vi "传感器特性判定.vi"(7 "Result":refnum<vi>, 10 "判定参数":T1, 11 "XY曲线":cluster{"X":dbl[], "Y":dbl[]}[](array[cluster])) -> (2 "判定项长度":i32, 3 "OK？":bool)   [LabVIEW 2020]
uses:
  <vilib>/Analysis/6fits.llb/Curve Fitting Criteria.ctl
  <vilib>/Analysis/NI_AALPro.lvlib
  <vilib>/Analysis/NI_AAL_Geometry.lvlib
panel:
  out "定点设置":dbl
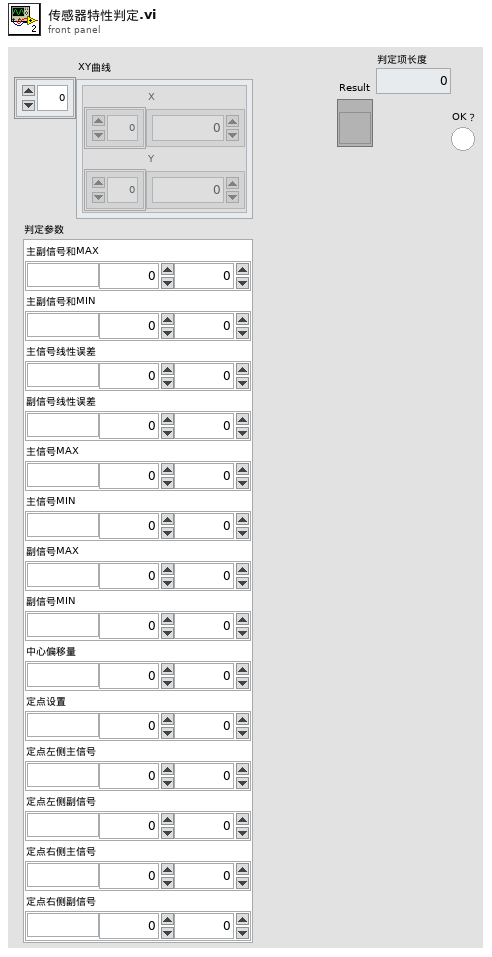
[diagram p1: front panel]
types:
  T1 = cluster{"主副信号和MAX":cluster{"单位":string, "下限":dbl, "上限":dbl}, "主副信号和MIN":cluster{"单位":string, "下限":dbl, "上限":dbl}, "主信号线性误差":cluster{"单位":string, "下限":dbl, "上限":dbl}, "副信号线性误差":cluster{"单位":string, "下限":dbl, "上限":dbl}, "主信号MAX":cluster{"单位":string, "下限":dbl, "上限":dbl}, "主信号MIN":cluster{"单位":string, "下限":dbl, "上限":dbl}, "副信号MAX":cluster{"单位":string, "下限":dbl, "上限":dbl}, "副信号MIN":cluster{"单位":string, "下限":dbl, "上限":dbl}, "中心偏移量":cluster{"单位":string, "下限":dbl, "上限":dbl}, "定点设置":cluster{"单位":string, "下限":dbl, "上限":dbl}, "定点左侧主信号":cluster{"单位":string, "下限":dbl, "上限":dbl}, "定点左侧副信号":cluster{"单位":string, "下限":dbl, "上限":dbl}, "定点右侧主信号":cluster{"单位":string, "下限":dbl, "上限":dbl}, "定点右侧副信号":cluster{"单位":string, "下限":dbl, "上限":dbl}}
  T2 = typedef "NI_AALPro.lvlib/Curve Fitting Criteria.ctl" = u16
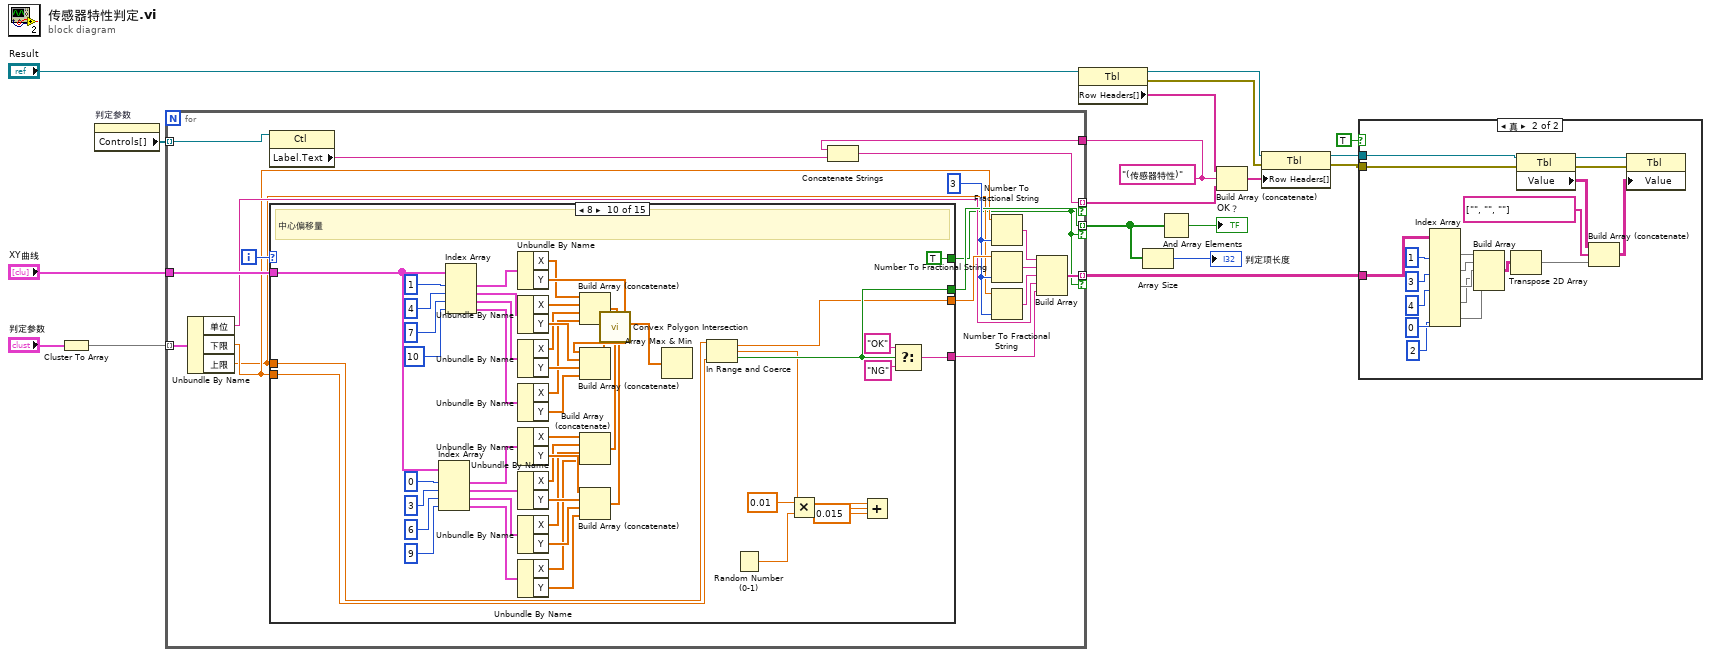
[diagram p0: block diagram]
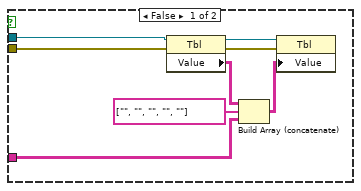
[diagram p2: hidden frame]
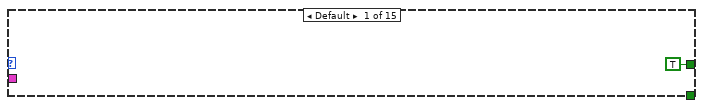
[diagram p3: hidden frame]
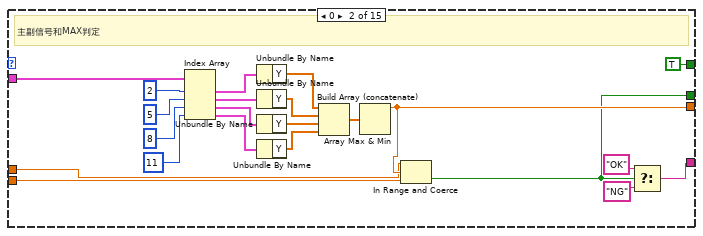
[diagram p4: hidden frame]
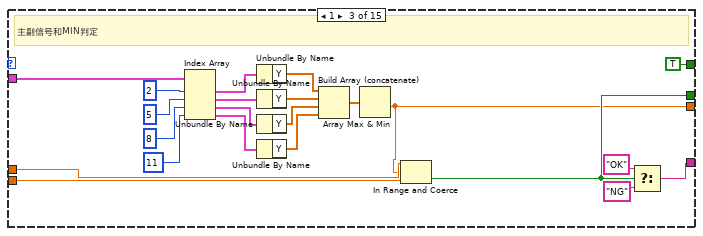
[diagram p5: hidden frame]
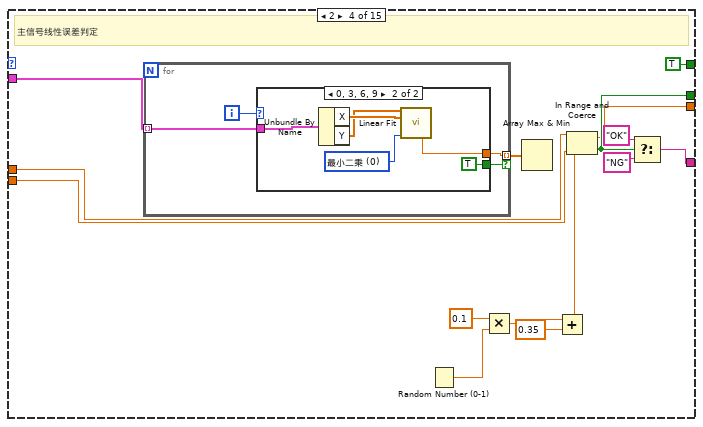
[diagram p6: hidden frame]
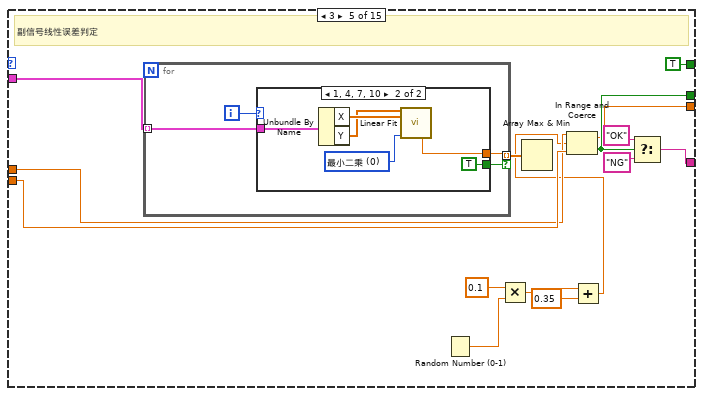
[diagram p8: hidden frame]
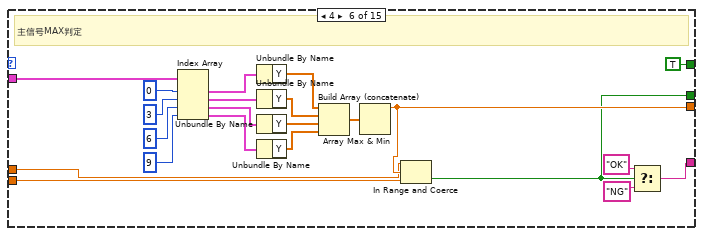
[diagram p10: hidden frame]
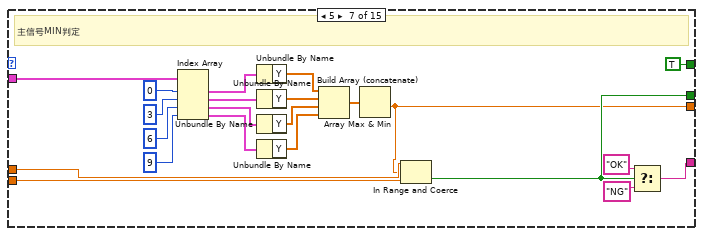
[diagram p11: hidden frame]
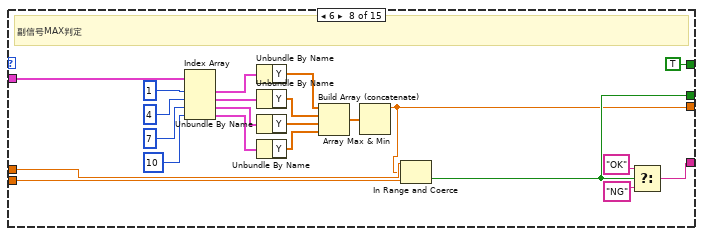
[diagram p12: hidden frame]
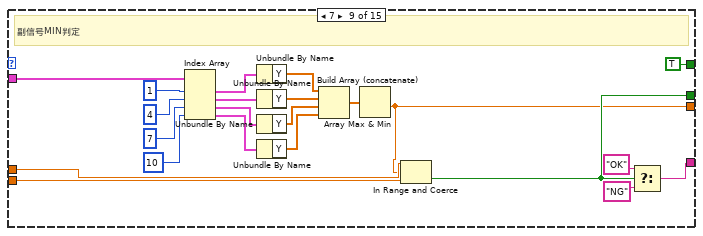
[diagram p13: hidden frame]
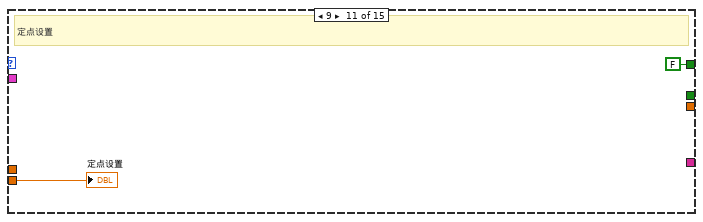
[diagram p14: hidden frame]
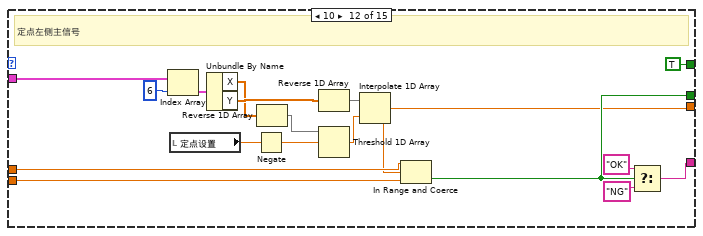
[diagram p15: hidden frame]
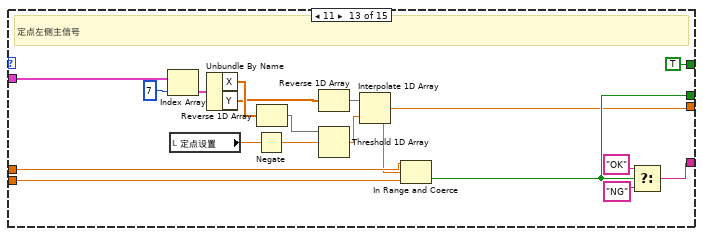
[diagram p16: hidden frame]
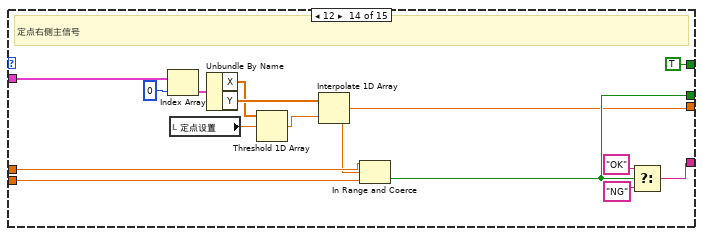
[diagram p17: hidden frame]
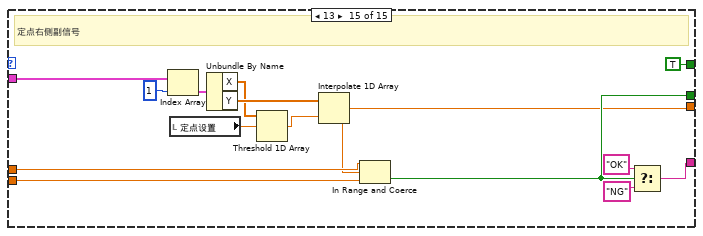
[diagram p18: hidden frame]
diagram:
  w1 = "(传感器特性)" ("Label.Text")
  n1 = Cluster To Array(cluster="判定参数") -> (array=w18:cluster{"单位":string, "下限":dbl, "上限":dbl}[])
  n2 = property on="判定参数" class="Clust (严格)"() -> ("Controls[]"=w16:refnum<vi>[])  [unwired: 2 in, 2 out]
  n3 = for {
    tunnel: w18 -> [w37] mode=indexing
    tunnel: w16 -> [w35] mode=indexing
    tunnel: "XY曲线" -> [w33]
    tunnel: [w27] -> w3 mode=indexing if=w21
    tunnel: [w23] -> w5 mode=indexing if=w21
    tunnel: [w20] -> w8 mode=indexing if=w21
    tunnel: w1 -> [w19]
    i -> [w36]
    w32 = i16 3 ("精度(6)")
    n4 = Unbundle By Name(w37) -> ("单位"=w26:string, "下限"=w25:dbl, "上限"=w24:dbl)
    n5 = property class="Ctl"(reference=w35) -> ("Label.Text"=w22:string)  [unwired: 1 in, 2 out]
    n6 = case shown="8" w36 {
      tunnel: [_ w46 w61 w84 w109 w140 w156 w178 w200 w222 _ w278 w295 w312 w327] -> w34
      tunnel: w33 -> [_ w60 w82 w90 w115 w154 w176 w198 w220 w240 _ w291 w309 w324 w339]
      tunnel: [_ w43 w66 w95 w120 w137 w160 w182 w204 w257 _ w287 w305 w320 w335] -> w28
      tunnel: [_ w42 w65 w94 w119 w136 w159 w181 w203 w256 _ w286 w304 w319 w334] -> w27
      tunnel: w25 -> [_ w41 w64 w93 w118 w135 w158 w180 w202 w255 w272 w285 w303 w318 w333]
      tunnel: w24 -> [_ w40 w63 w92 w117 w134 w157 w179 w201 w254 _ w284 w302 w317 w332]
      tunnel: [TRUE TRUE TRUE TRUE TRUE TRUE TRUE TRUE TRUE TRUE FALSE TRUE TRUE TRUE TRUE] -> w21
      frame Default {
      }
      frame 0 {
        # "主副信号和MAX判定"
        n7 = Index Array(array=w60, index #1=2 ("索引"), index #2=5 ("索引"), index #3=8 ("索引"), index #4=11 ("索引")) -> (element #1=w55:cluster{"X":dbl[], "Y":dbl[]}, element #2=w52:cluster{"X":dbl[], "Y":dbl[]}, element #3=w53:cluster{"X":dbl[], "Y":dbl[]}, element #4=w54:cluster{"X":dbl[], "Y":dbl[]})
        n8 = Unbundle By Name(w55) -> ("Y"=w51:dbl[])
        n9 = Unbundle By Name(w52) -> ("Y"=w50:dbl[])
        n10 = Unbundle By Name(w53) -> ("Y"=w49:dbl[])
        n11 = Unbundle By Name(w54) -> ("Y"=w48:dbl[])
        n12 = Build Array (concatenate)(w51, w50, w49, w48) -> (w47:dbl[])
        n13 = Array Max & Min(array=w47) -> (max value=w46:dbl)  [unwired: 3 out]
        n14 = In Range and Coerce(upper limit=w40, x=w46, lower limit=w41) -> (In Range?=w42:bool)  [unwired: 1 out]
        n15 = Select(t="OK", s=w42, f="NG") -> (s? t:f=w43:string)
      }
      frame 1 {
        # "主副信号和MIN判定"
        n16 = Index Array(array=w82, index #1=2 ("索引"), index #2=5 ("索引"), index #3=8 ("索引"), index #4=11 ("索引")) -> (element #1=w77:cluster{"X":dbl[], "Y":dbl[]}, element #2=w74:cluster{"X":dbl[], "Y":dbl[]}, element #3=w75:cluster{"X":dbl[], "Y":dbl[]}, element #4=w76:cluster{"X":dbl[], "Y":dbl[]})
        n17 = Unbundle By Name(w77) -> ("Y"=w73:dbl[])
        n18 = Unbundle By Name(w74) -> ("Y"=w72:dbl[])
        n19 = Unbundle By Name(w75) -> ("Y"=w71:dbl[])
        n20 = Unbundle By Name(w76) -> ("Y"=w70:dbl[])
        n21 = Build Array (concatenate)(w73, w72, w71, w70) -> (w69:dbl[])
        n22 = Array Max & Min(array=w69) -> (min value=w61:dbl)  [unwired: 3 out]
        n23 = In Range and Coerce(upper limit=w63, x=w61, lower limit=w64) -> (In Range?=w65:bool)  [unwired: 1 out]
        n24 = Select(t="OK", s=w65, f="NG") -> (s? t:f=w66:string)
      }
      frame 2 {
        # "主信号线性误差判定"
        n25 = for {
          tunnel: w90 -> [w100] mode=indexing
          tunnel: [w99] -> w89 mode=indexing if=w98
          i -> [w101]
          n26 = case shown="0, 3, 6, 9" w101 {
            tunnel: w100 -> [_ w107]
            tunnel: [_ w105] -> w99
            tunnel: [_ TRUE] -> w98
            frame Default {
            }
            frame 0, 3, 6, 9 {
              w106 = T2 0 items=["最小二乘", "最小绝对残差", "Bisquare"] ("method")
              n27 = Unbundle By Name(w107) -> ("X"=w103:dbl[], "Y"=w102:dbl[])
              n28 = call <vilib>:"Linear Fit.vi"("Y"=w102, "X"=w103, "method"=w106) -> ("residue"=w105:dbl)  [unwired: 8 in, 4 out]
            }
          }
        }
        n29 = Random Number (0-1)() -> (number: 0 to 1=w87:dbl)
        n30 = Multiply(x=0.1, y=w87) -> (x*y=w86:dbl)
        n31 = Array Max & Min(array=w89) -> ()  [unwired: 4 out]
        n32 = Add(x=w86, y=0.35) -> (x+y=w83:dbl)
        n33 = In Range and Coerce(upper limit=w92, x=w83, lower limit=w93) -> (coerced(x)=w84:dbl, In Range?=w94:bool)
        n34 = Select(t="OK", s=w94, f="NG") -> (s? t:f=w95:string)
      }
      frame 3 {
        # "副信号线性误差判定"
        n35 = for {
          tunnel: w115 -> [w125] mode=indexing
          tunnel: [w124] -> w114 mode=indexing if=w123
          i -> [w126]
          n36 = case shown="1, 4, 7, 10" w126 {
            tunnel: w125 -> [_ w132]
            tunnel: [_ w130] -> w124
            tunnel: [_ TRUE] -> w123
            frame Default {
            }
            frame 1, 4, 7, 10 {
              w131 = T2 0 items=["最小二乘", "最小绝对残差", "Bisquare"] ("method")
              n37 = Unbundle By Name(w132) -> ("X"=w128:dbl[], "Y"=w127:dbl[])
              n38 = call <vilib>:"Linear Fit.vi"("Y"=w127, "X"=w128, "method"=w131) -> ("residue"=w130:dbl)  [unwired: 8 in, 4 out]
            }
          }
        }
        n39 = Random Number (0-1)() -> (number: 0 to 1=w113:dbl)
        n40 = Multiply(x=0.1, y=w113) -> (x*y=w112:dbl)
        n41 = Array Max & Min(array=w114) -> ()  [unwired: 4 out]
        n42 = Add(x=w112, y=0.35) -> (x+y=w108:dbl)
        n43 = In Range and Coerce(upper limit=w117, x=w108, lower limit=w118) -> (coerced(x)=w109:dbl, In Range?=w119:bool)
        n44 = Select(t="OK", s=w119, f="NG") -> (s? t:f=w120:string)
      }
      frame 4 {
        # "主信号MAX判定"
        n45 = Index Array(array=w154, index #1=0 ("索引"), index #2=3 ("索引"), index #3=6 ("索引"), index #4=9 ("索引")) -> (element #1=w149:cluster{"X":dbl[], "Y":dbl[]}, element #2=w146:cluster{"X":dbl[], "Y":dbl[]}, element #3=w147:cluster{"X":dbl[], "Y":dbl[]}, element #4=w148:cluster{"X":dbl[], "Y":dbl[]})
        n46 = Unbundle By Name(w149) -> ("Y"=w145:dbl[])
        n47 = Unbundle By Name(w146) -> ("Y"=w144:dbl[])
        n48 = Unbundle By Name(w147) -> ("Y"=w143:dbl[])
        n49 = Unbundle By Name(w148) -> ("Y"=w142:dbl[])
        n50 = Build Array (concatenate)(w145, w144, w143, w142) -> (w141:dbl[])
        n51 = Array Max & Min(array=w141) -> (max value=w140:dbl)  [unwired: 3 out]
        n52 = In Range and Coerce(upper limit=w134, x=w140, lower limit=w135) -> (In Range?=w136:bool)  [unwired: 1 out]
        n53 = Select(t="OK", s=w136, f="NG") -> (s? t:f=w137:string)
      }
      frame 5 {
        # "主信号MIN判定"
        n54 = Index Array(array=w176, index #1=0 ("索引"), index #2=3 ("索引"), index #3=6 ("索引"), index #4=9 ("索引")) -> (element #1=w171:cluster{"X":dbl[], "Y":dbl[]}, element #2=w168:cluster{"X":dbl[], "Y":dbl[]}, element #3=w169:cluster{"X":dbl[], "Y":dbl[]}, element #4=w170:cluster{"X":dbl[], "Y":dbl[]})
        n55 = Unbundle By Name(w171) -> ("Y"=w167:dbl[])
        n56 = Unbundle By Name(w168) -> ("Y"=w166:dbl[])
        n57 = Unbundle By Name(w169) -> ("Y"=w165:dbl[])
        n58 = Unbundle By Name(w170) -> ("Y"=w164:dbl[])
        n59 = Build Array (concatenate)(w167, w166, w165, w164) -> (w163:dbl[])
        n60 = Array Max & Min(array=w163) -> (min value=w156:dbl)  [unwired: 3 out]
        n61 = In Range and Coerce(upper limit=w157, x=w156, lower limit=w158) -> (In Range?=w159:bool)  [unwired: 1 out]
        n62 = Select(t="OK", s=w159, f="NG") -> (s? t:f=w160:string)
      }
      frame 6 {
        # "副信号MAX判定"
        n63 = Index Array(array=w198, index #1=1 ("索引"), index #2=4 ("索引"), index #3=7 ("索引"), index #4=10 ("索引")) -> (element #1=w193:cluster{"X":dbl[], "Y":dbl[]}, element #2=w190:cluster{"X":dbl[], "Y":dbl[]}, element #3=w191:cluster{"X":dbl[], "Y":dbl[]}, element #4=w192:cluster{"X":dbl[], "Y":dbl[]})
        n64 = Unbundle By Name(w193) -> ("Y"=w189:dbl[])
        n65 = Unbundle By Name(w190) -> ("Y"=w188:dbl[])
        n66 = Unbundle By Name(w191) -> ("Y"=w187:dbl[])
        n67 = Unbundle By Name(w192) -> ("Y"=w186:dbl[])
        n68 = Build Array (concatenate)(w189, w188, w187, w186) -> (w185:dbl[])
        n69 = Array Max & Min(array=w185) -> (max value=w178:dbl)  [unwired: 3 out]
        n70 = In Range and Coerce(upper limit=w179, x=w178, lower limit=w180) -> (In Range?=w181:bool)  [unwired: 1 out]
        n71 = Select(t="OK", s=w181, f="NG") -> (s? t:f=w182:string)
      }
      frame 7 {
        # "副信号MIN判定"
        n72 = Index Array(array=w220, index #1=1 ("索引"), index #2=4 ("索引"), index #3=7 ("索引"), index #4=10 ("索引")) -> (element #1=w215:cluster{"X":dbl[], "Y":dbl[]}, element #2=w212:cluster{"X":dbl[], "Y":dbl[]}, element #3=w213:cluster{"X":dbl[], "Y":dbl[]}, element #4=w214:cluster{"X":dbl[], "Y":dbl[]})
        n73 = Unbundle By Name(w215) -> ("Y"=w211:dbl[])
        n74 = Unbundle By Name(w212) -> ("Y"=w210:dbl[])
        n75 = Unbundle By Name(w213) -> ("Y"=w209:dbl[])
        n76 = Unbundle By Name(w214) -> ("Y"=w208:dbl[])
        n77 = Build Array (concatenate)(w211, w210, w209, w208) -> (w207:dbl[])
        n78 = Array Max & Min(array=w207) -> (min value=w200:dbl)  [unwired: 3 out]
        n79 = In Range and Coerce(upper limit=w201, x=w200, lower limit=w202) -> (In Range?=w203:bool)  [unwired: 1 out]
        n80 = Select(t="OK", s=w203, f="NG") -> (s? t:f=w204:string)
      }
      frame 8 {
        # "中心偏移量"
        n81 = Index Array(array=w240, index #1=0 ("索引"), index #2=3 ("索引"), index #3=6 ("索引"), index #4=9 ("索引")) -> (element #1=w267:cluster{"X":dbl[], "Y":dbl[]}, element #2=w264:cluster{"X":dbl[], "Y":dbl[]}, element #3=w265:cluster{"X":dbl[], "Y":dbl[]}, element #4=w266:cluster{"X":dbl[], "Y":dbl[]})
        n82 = Index Array(array=w240, index #1=1 ("索引"), index #2=4 ("索引"), index #3=7 ("索引"), index #4=10 ("索引")) -> (element #1=w245:cluster{"X":dbl[], "Y":dbl[]}, element #2=w248:cluster{"X":dbl[], "Y":dbl[]}, element #3=w247:cluster{"X":dbl[], "Y":dbl[]}, element #4=w246:cluster{"X":dbl[], "Y":dbl[]})
        n83 = Unbundle By Name(w245) -> ("X"=w239:dbl[], "Y"=w249:dbl[])
        n84 = Unbundle By Name(w248) -> ("X"=w238:dbl[], "Y"=w250:dbl[])
        n85 = Unbundle By Name(w247) -> ("X"=w237:dbl[], "Y"=w251:dbl[])
        n86 = Unbundle By Name(w246) -> ("X"=w236:dbl[], "Y"=w252:dbl[])
        n87 = Unbundle By Name(w267) -> ("X"=w235:dbl[], "Y"=w263:dbl[])
        n88 = Unbundle By Name(w264) -> ("X"=w234:dbl[], "Y"=w262:dbl[])
        n89 = Unbundle By Name(w265) -> ("X"=w233:dbl[], "Y"=w261:dbl[])
        n90 = Unbundle By Name(w266) -> ("X"=w232:dbl[], "Y"=w260:dbl[])
        n91 = Build Array (concatenate)(w239, w238, w237, w236) -> (w229:dbl[])
        n92 = Build Array (concatenate)(w249, w250, w251, w252) -> (w231:dbl[])
        n93 = Build Array (concatenate)(w235, w234, w233, w232) -> (w228:dbl[])
        n94 = Build Array (concatenate)(w263, w262, w261, w260) -> (w227:dbl[])
        n95 = call <vilib>:"Convex Polygon Intersection.vi"("Y 2"=w227, "X 2"=w228, "Y 1"=w231, "X 1"=w229) -> ("Intersection Y"=w230:dbl[])  [unwired: 5 in, 2 out]
        n96 = Array Max & Min(array=w230) -> ()  [unwired: 4 out]
        n97 = Random Number (0-1)() -> (number: 0 to 1=w225:dbl)
        n98 = Multiply(x=0.01, y=w225) -> (x*y=w224:dbl)
        n99 = Add(x=w224, y=0.015) -> (x+y=w221:dbl)
        n100 = In Range and Coerce(upper limit=w254, x=w221, lower limit=w255) -> (coerced(x)=w222:dbl, In Range?=w256:bool)
        n101 = Select(t="OK", s=w256, f="NG") -> (s? t:f=w257:string)
      }
      frame 9 {
        # "定点设置"
        "定点设置" <- w272
      }
      frame 10 {
        # "定点左侧主信号"
        n102 = Index Array(array=w291, index=6 ("索引")) -> (element=w290:cluster{"X":dbl[], "Y":dbl[]})
        n103 = local read "定点设置"() -> (w280:dbl)
        n104 = Unbundle By Name(w290) -> ("X"=w277:dbl[], "Y"=w279:dbl[])
        n105 = Negate(x=w280) -> (-x=w276:dbl)
        n106 = Reverse 1D Array(array=w277) -> (reversed array=w275:dbl[])
        n107 = Reverse 1D Array(array=w279) -> (reversed array=w274:dbl[])
        n108 = Threshold 1D Array(2:w276, 3:w275) -> (0:w281:dbl)  [unwired: 1 in]
        n109 = Interpolate 1D Array(1:w281, 2:w274) -> (0:w278:dbl)
        n110 = In Range and Coerce(upper limit=w284, x=w278, lower limit=w285) -> (In Range?=w286:bool)  [unwired: 1 out]
        n111 = Select(t="OK", s=w286, f="NG") -> (s? t:f=w287:string)
      }
      frame 11 {
        # "定点左侧主信号"
        n112 = Index Array(array=w309, index=7 ("索引")) -> (element=w308:cluster{"X":dbl[], "Y":dbl[]})
        n113 = local read "定点设置"() -> (w297:dbl)
        n114 = Unbundle By Name(w308) -> ("X"=w298:dbl[], "Y"=w296:dbl[])
        n115 = Negate(x=w297) -> (-x=w292:dbl)
        n116 = Reverse 1D Array(array=w298) -> (reversed array=w294:dbl[])
        n117 = Reverse 1D Array(array=w296) -> (reversed array=w293:dbl[])
        n118 = Threshold 1D Array(2:w292, 3:w294) -> (0:w299:dbl)  [unwired: 1 in]
        n119 = Interpolate 1D Array(1:w299, 2:w293) -> (0:w295:dbl)
        n120 = In Range and Coerce(upper limit=w302, x=w295, lower limit=w303) -> (In Range?=w304:bool)  [unwired: 1 out]
        n121 = Select(t="OK", s=w304, f="NG") -> (s? t:f=w305:string)
      }
      frame 12 {
        # "定点右侧主信号"
        n122 = Index Array(array=w324, index=0 ("索引")) -> (element=w323:cluster{"X":dbl[], "Y":dbl[]})
        n123 = local read "定点设置"() -> (w310:dbl)
        n124 = Unbundle By Name(w323) -> ("X"=w311:dbl[], "Y"=w313:dbl[])
        n125 = Threshold 1D Array(2:w310, 3:w311) -> (0:w314:dbl)  [unwired: 1 in]
        n126 = Interpolate 1D Array(1:w314, 2:w313) -> (0:w312:dbl)
        n127 = In Range and Coerce(upper limit=w317, x=w312, lower limit=w318) -> (In Range?=w319:bool)  [unwired: 1 out]
        n128 = Select(t="OK", s=w319, f="NG") -> (s? t:f=w320:string)
      }
      frame 13 {
        # "定点右侧副信号"
        n129 = Index Array(array=w339, index=1 ("索引")) -> (element=w338:cluster{"X":dbl[], "Y":dbl[]})
        n130 = local read "定点设置"() -> (w325:dbl)
        n131 = Unbundle By Name(w338) -> ("X"=w326:dbl[], "Y"=w328:dbl[])
        n132 = Threshold 1D Array(2:w325, 3:w326) -> (0:w329:dbl)  [unwired: 1 in]
        n133 = Interpolate 1D Array(1:w329, 2:w328) -> (0:w327:dbl)
        n134 = In Range and Coerce(upper limit=w332, x=w327, lower limit=w333) -> (In Range?=w334:bool)  [unwired: 1 out]
        n135 = Select(t="OK", s=w334, f="NG") -> (s? t:f=w335:string)
      }
    }
    n136 = Concatenate Strings(w19, w22) -> (w20:string)
    n137 = Number To Fractional String(number=w25, precision (6)=w32) -> (F-format string=w31:string)  [unwired: 2 in]
    n138 = Number To Fractional String(number=w34, precision (6)=w32) -> (F-format string=w30:string)  [unwired: 2 in]
    n139 = Number To Fractional String(number=w24, precision (6)=w32) -> (F-format string=w29:string)  [unwired: 2 in]
    n140 = Build Array(w31, w30, w29, w26, w28) -> (w23:string[])
  }
  n141 = property class="Tbl"(reference="Result") -> (reference out=w10:refnum<vi>, error out=w13:errorcluster, "Row Headers[]"=w6:string[])  [unwired: 1 in]
  n142 = Array Size(array=w3) -> (size(s)=→"判定项长度":i32)
  n143 = And Array Elements(Boolean array=w3) -> (logical AND=→"OK？":bool)
  n144 = Build Array (concatenate)(w6, w1, w8) -> (w9:string[])
  n145 = property class="Tbl"(reference=w10, error in=w13, "Row Headers[]"=w9) -> (reference out=w11:refnum<vi>, error out=w12:errorcluster)
  n146 = case shown="真" TRUE {
    tunnel: w12 -> [w345 w365]
    tunnel: w11 -> [w342 w362]
    tunnel: w5 -> [w341 w353]
    frame False {
      n147 = property class="Tbl"(reference=w342, error in=w345) -> (reference out=w343:refnum<vi>, error out=w344:errorcluster, "Value"=w346:string[][])
      n148 = Build Array (concatenate)(w346, string[] ["", "", "", "", ""], w341) -> (w347:string[][])
      n149 = property class="Tbl"(reference=w343, error in=w344, "Value"=w347) -> ()  [unwired: 2 out]
    }
    frame True {
      n150 = Index Array(array=w353, index (col) #1=1 ("禁用的索引 (列)"), index (col) #2=3 ("索引 (列)"), index (col) #3=4 ("索引 (列)"), index (col) #4=0 ("索引 (列)"), index (col) #5=2 ("索引 (列)")) -> (element #1=w357:string[], element #2=w356:string[], element #3=w355:string[], element #4=w349:string[], element #5=w348:string[])  [unwired: 5 in]
      n151 = Build Array(w357, w356, w355, w349, w348) -> (w354:string[][])
      n152 = Transpose 2D Array(2D array=w354) -> (transposed array=w352:string[][])
      n153 = property class="Tbl"(reference=w362, error in=w365) -> (reference out=w363:refnum<vi>, error out=w364:errorcluster, "Value"=w366:string[][])
      n154 = Build Array (concatenate)(w366, string[] ["", "", ""], w352) -> (w367:string[][])
      n155 = property class="Tbl"(reference=w363, error in=w364, "Value"=w367) -> ()  [unwired: 2 out]
    }
  }
